vi "ElevEncActions.vi"(10 "Update?":bool, 11 "Zero?":bool) -> (3 "ElevEncPos":i32)   [LabVIEW 2018]
uses:
  <vilib>/Rock Robotics/WPI/ThirdParty/Phoenix-LabVIEW/Motor Controller/Get/CTRE_Phoenix_MotorController_GetQuadratureData.vi
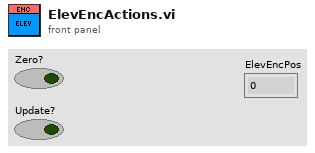
[diagram p1: front panel]
types:
  T1 = typedef "WPI_MotorControlDeviceRef.ctl" = cluster{"DeviceStatus":errorcluster, "Type":T2, "PWM":cluster{"PWM Channel":T3, "DeadBand":T4}, "CAN":cluster{"Device Number":u8, "SetOutput VI Ref":variant, "GetOutput VI Ref":variant, "Enable VI Ref":variant, "Disable VI Ref":variant, "Data":variant}, "Invert":bool, "DIO PWM":cluster{"PWM \"Enable\" Channel":T3, "DIOChannel":T5, "PWM Rate":dbl}}
  T2 = typedef "WPI_MotorControlType.ctl" = enum16{"PWM", "CAN", "DIO PWM"}
  T3 = typedef "FPGA_DIOPWMChannel.ctl" = enum8{"PWM 0", "PWM 1", "PWM 2", "PWM 3", "PWM 4", "PWM 5", "PWM 6", "PWM 7", "PWM 8", "PWM 9", "PWM MXP 0", "PWM MXP 1", "PWM MXP 2", "PWM MXP 3", "PWM MXP 4", "PWM MXP 5", "PWM MXP 6", "PWM MXP 7", "PWM MXP 8", "PWM MXP 9", "Invalid"}
  T4 = typedef "WPI_PWMDeadband.ctl" = cluster{"Name":string, "maxPositivePwm":i32, "minPositivePwm":i32, "centerPwm":i32, "maxNegativePwm":i32, "minNegativePwm":i32, "angularRange":u16}
  T5 = typedef "FPGA_DIOChannel.ctl" = enum8{"DIO 0", "DIO 1", "DIO 2", "DIO 3", "DIO 4", "DIO 5", "DIO 6", "DIO 7", "DIO 8", "DIO 9", "DIO MXP 0", "DIO MXP 1", "DIO MXP 2", "DIO MXP 3", "DIO MXP 4", "DIO MXP 5", "DIO MXP 6", "DIO MXP 7", "DIO MXP 8", "DIO MXP 9", "DIO MXP 10", "DIO MXP 11", "DIO MXP 12", "DIO MXP 13", "DIO MXP 14", "DIO MXP 15", "SPI Port CS1", "SPI Port CS2", "SPI Port CS3", "SPI Port MISO", "SPI Port MOSI", "Invalid"}
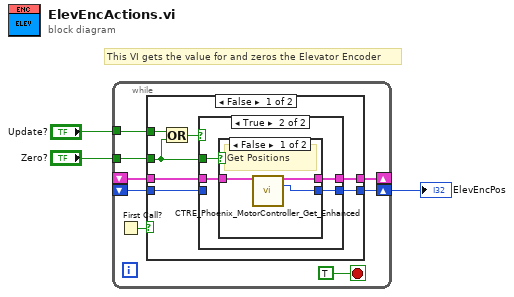
[diagram p0: block diagram]
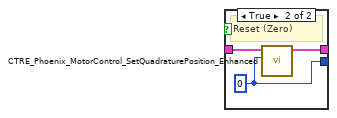
[diagram p3: hidden frame]
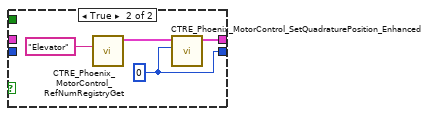
[diagram p4: hidden frame]
diagram:
  # "This VI gets the value for and zeros the Elevator Encoder"
  n1 = while {
    shift-right: [w10] -> _
    shift-left: _ -> [w9]
    tunnel: "Zero?" -> [w6]
    tunnel: "Update?" -> [w5]
    shift-right: [w11] -> w1
    shift-left: _ -> [w4]
    stop <- TRUE stop-if-true
    n2 = First Call?() -> (First Call?: T/F=w8:bool)
    n3 = case shown="False" w8 {
      tunnel: w9 -> [w18 _]
      tunnel: [w17 w31] -> w11
      tunnel: [w16 w32] -> w10
      tunnel: w6 -> [w12 _]
      tunnel: w5 -> [w13 _]
      tunnel: w4 -> [w14 _]
      frame False {
        n4 = Or(x=w13, y=w12) -> (x .or. y?=w15:bool)
        n5 = case shown="True" w15 {
          tunnel: w18 -> [w20 w24]
          tunnel: [w19 w23] -> w17
          tunnel: [w20 w22] -> w16
          tunnel: w12 -> [_ w21]
          tunnel: w14 -> [w19 _]
          frame False {
          }
          frame True {
            n6 = case shown="False" w21 {
              tunnel: w24 -> [w27 w30]
              tunnel: [w26 w28] -> w23
              tunnel: [w25 w29] -> w22
              frame False {
                # "Get Positions"
                n7 = call-poly <vilib>:"CTRE_Phoenix_MotorController_Get_Enhanced.vi"("PhoenixMotorControlDevRef"=w27) -> ("PhoenixMotorControlDevRef"=w25:T1, "Quadrature Position"=w26:i32)  [unwired: 11 in, 2 out]
              }
              frame True {
                w28 = 0 ("New Position")
                # "Reset (Zero)"
                n8 = call <vilib>:"CTRE_Phoenix_MotorControl_SetQuadraturePosition_Enhanced.vi"("New Position"=w28, "PhoenixMotorControlDevRef"=w30) -> ("PhoenixMotorControlDevRef"=w29:T1)  [unwired: 8 in, 1 out]
              }
            }
          }
        }
      }
      frame True {
        w31 = 0 ("New Sensor Position")
        n9 = call <vilib>:"CTRE_Phoenix_MotorControl_RefNumRegistryGet.vi"("refnum name"="Elevator") -> ("PhoenixMotorControlDevRef"=w33:T1)  [unwired: 9 in, 1 out]
        n10 = call <vilib>:"CTRE_Phoenix_MotorControl_SetQuadraturePosition_Enhanced.vi"("New Position"=w31, "PhoenixMotorControlDevRef"=w33) -> ("PhoenixMotorControlDevRef"=w32:T1)  [unwired: 8 in, 1 out]
      }
    }
  }
  "ElevEncPos" <- w1
